vi "bootfile.vi"(11 "parameter file":path=path "D:/dsp files/base_config.set") -> ()   [LabVIEW 2016]
doc: "bootfile.VI connects to the Pixie4 and loads the chosen DSP file. Due to PRIME Lab using 2 PXI crates, the crate size and slot # will need to be adjusted to attain the proper PCI bus address."
uses:
  controls/pixie crates.ctl
  bootfile states.ctl
panel:
  in  "Select PXI chassis type":T1=enum."18-slot chassis"
  in  "Total number of Pixie-4 modules":u16=1
  in  "Slot(s) of Pixie4":u16[](array[numeric])=[8]
  in  "Set":bool
  # "2017.06.01 Note: The Pixie4 is in slot 3 of an 8-slot chassis, but PRIME Lab uses two PXI crates daisy-chained together and XIA's Pixie_Scan_Crate_Slots can't handle multi-crate systems.  Slot 8 of an 18-slot chassis has the same PCI bus and device numbers as Slot 3 of the 1st crate of a two PXI-crate system."
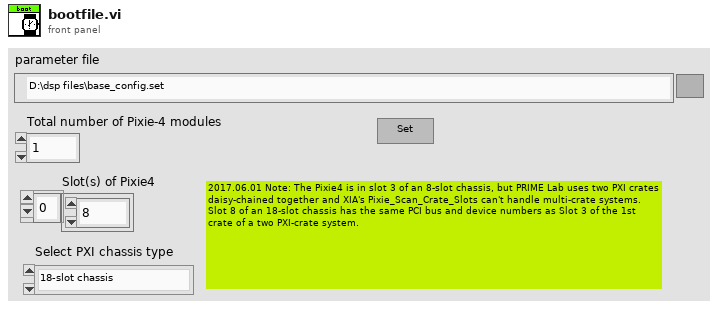
[diagram p1: front panel]
types:
  T1 = typedef "pixie crates.ctl" = enum16{"4 or 8-slot chassis", "14-slot chassis", "18-slot chassis"}
  T2 = typedef "bootfile states.ctl" = enum16{"wait", "set", "stop"}
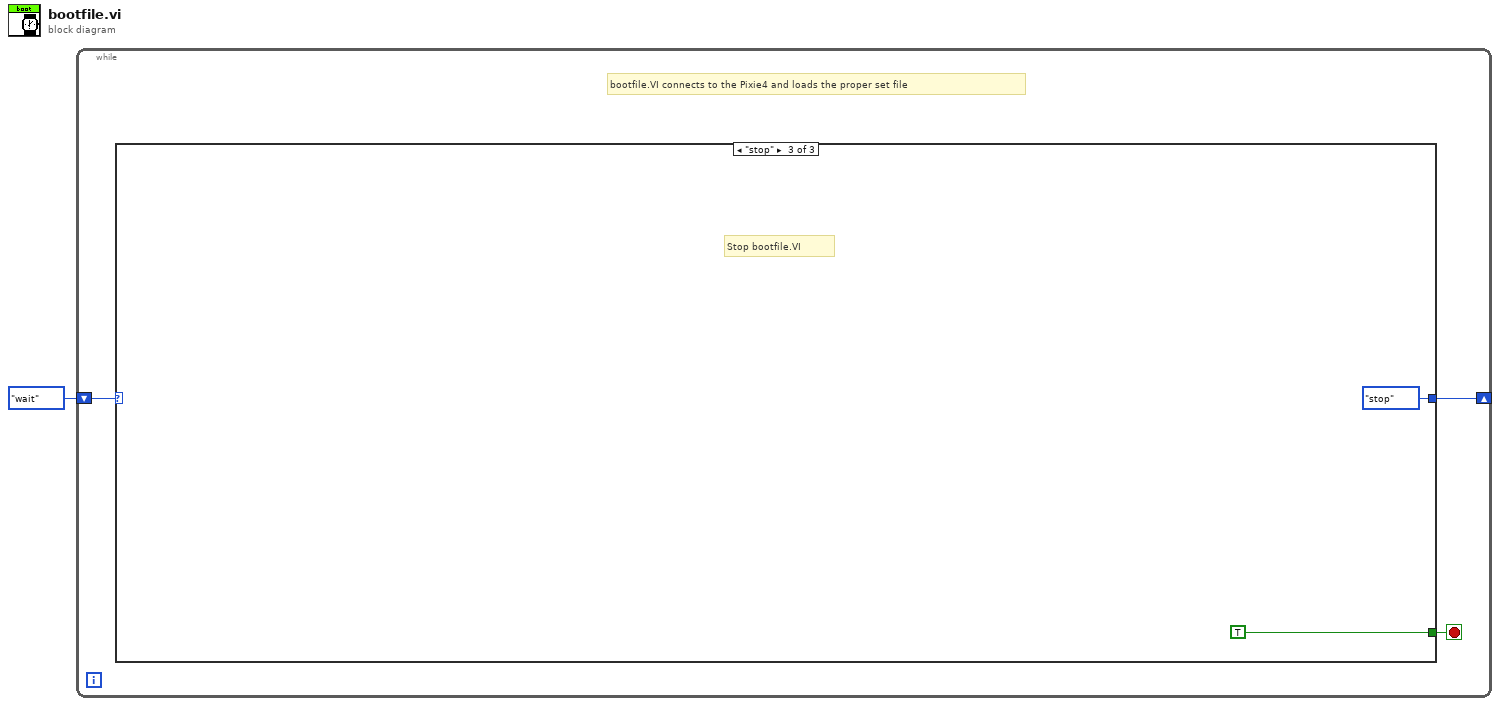
[diagram p0: block diagram]
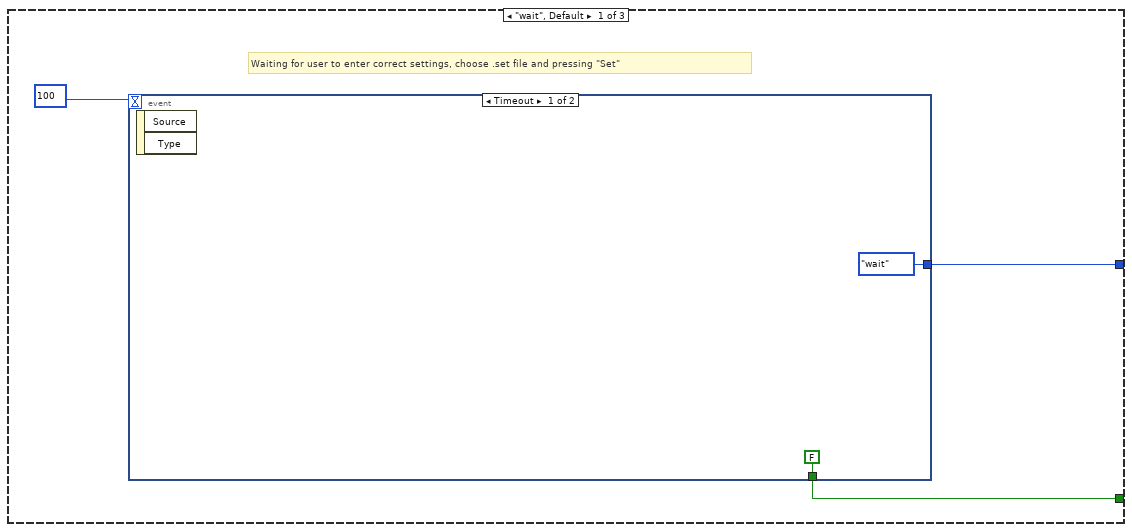
[diagram p2: hidden frame]
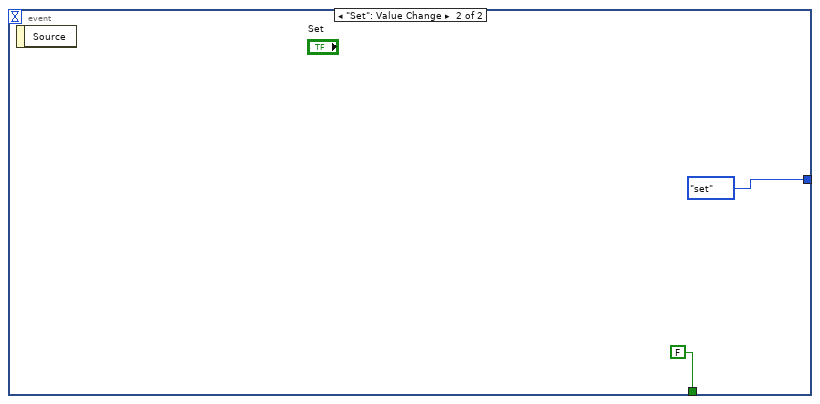
[diagram p3: hidden frame]
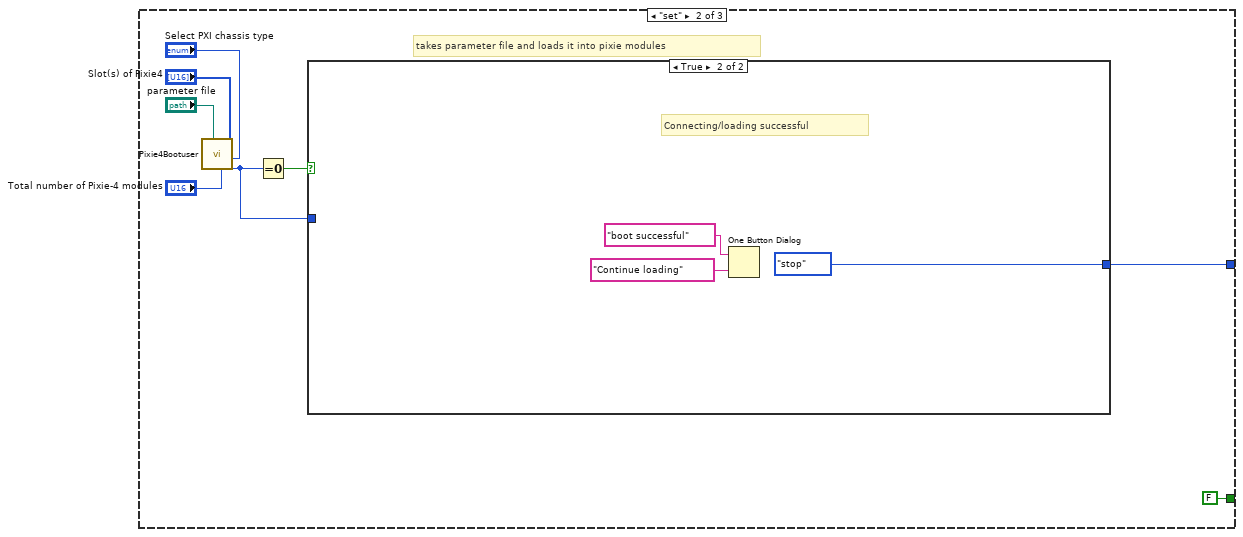
[diagram p4: hidden frame]
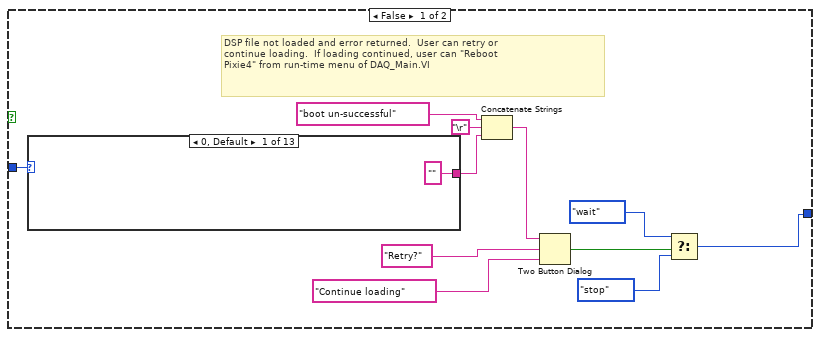
[diagram p5: hidden frame]
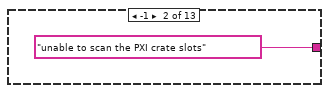
[diagram p6: hidden frame]
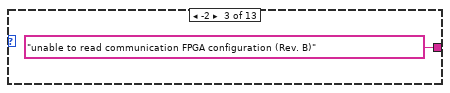
[diagram p7: hidden frame]
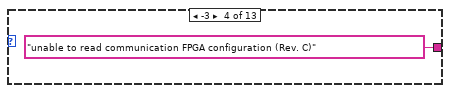
[diagram p8: hidden frame]
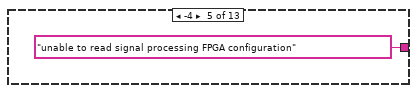
[diagram p9: hidden frame]
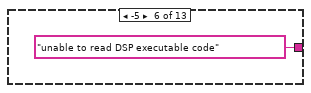
[diagram p10: hidden frame]
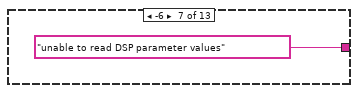
[diagram p11: hidden frame]
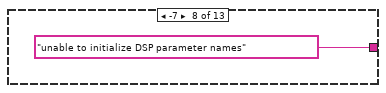
[diagram p12: hidden frame]
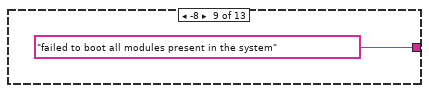
[diagram p13: hidden frame]
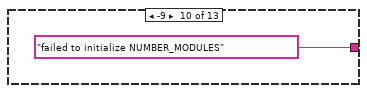
[diagram p14: hidden frame]
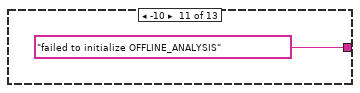
[diagram p15: hidden frame]
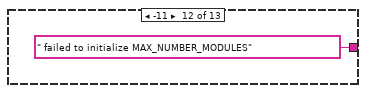
[diagram p16: hidden frame]
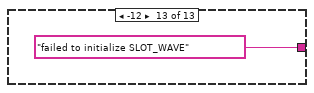
[diagram p17: hidden frame]
diagram:
  n1 = while {
    shift-right: [w2] -> _
    shift-left: bootfile_states."wait" -> [w3]
    stop <- w4 stop-if-true
    # "bootfile.VI connects to the Pixie4 and loads the proper set file"
    n2 = case shown="\"stop\"" w3 {
      tunnel: [w7 FALSE TRUE] -> w4
      tunnel: [w6 w14 bootfile_states."stop"] -> w2
      frame "wait", Default {
        # "Waiting for user to enter correct settings, choose .set file and pressing \"Set\""
        n3 = event shown="[0] Timeout" {
          selector: _ -> [_ _]
          dyn-events: _ -> [_ _]
          timeout: 100 -> [_ _]
          tunnel: [FALSE FALSE] -> w7
          tunnel: [bootfile_states."wait" bootfile_states."set"] -> w6
          event Timeout {
            n4 = event-data() -> ()  [unwired: 1 in, 2 out]
          }
          event "Set": Value Change {
            n5 = event-data() -> ()  [unwired: 1 in, 1 out]
          }
        }
      }
      frame "set" {
        # "takes parameter file and loads it into pixie modules"
        n6 = call "Pixie4Bootuser.vi"("Select PXI chassis type"="Select PXI chassis type", "Module #"="Slot(s) of Pixie4", "Total number of Pixie-4 modules"="Total number of Pixie-4 modules", "DSP parameters file (.set file in folder \"Configuration\")"="parameter file") -> ("Return value for booting"=w13:i32)  [unwired: 7 in]
        n7 = Equal To 0?(x=w13) -> (x = 0?=w15:bool)
        n8 = case shown="True" w15 {
          tunnel: [w22 bootfile_states."stop"] -> w14
          tunnel: w13 -> [w27 _]
          frame False {
            # "DSP file not loaded and error returned.  User can retry or \ncontinue loading.  If loading continued, user can \"Reboot\nPixie4\" from run-time menu of DAQ_Main.VI"
            n9 = case shown="0, Default" w27 {
              tunnel: ["" ("format string") "unable to scan the PXI crate slots" ("format string") "unable to read communication FPGA configuration (Rev. B)" ("format string") "unable to read communication FPGA configuration (Rev. C)" ("format string") "unable to read signal processing FPGA configuration" ("format string") "unable to read DSP executable code" ("format string") "unable to read DSP parameter values" ("format string") "unable to initialize DSP parameter names" ("format string") "failed to boot all modules present in the system" ("format string") "failed to initialize NUMBER_MODULES" ("format string") "failed to initialize OFFLINE_ANALYSIS" ("format string") " failed to initialize MAX_NUMBER_MODULES" ("format string") "failed to initialize SLOT_WAVE" ("format string")] -> w28
              frame 0, Default {
              }
              frame -1 {
              }
              frame -2 {
              }
              frame -3 {
              }
              frame -4 {
              }
              frame -5 {
              }
              frame -6 {
              }
              frame -7 {
              }
              frame -8 {
              }
              frame -9 {
              }
              frame -10 {
              }
              frame -11 {
              }
              frame -12 {
              }
            }
            n10 = Concatenate Strings("boot un-successful" ("format string"), "\r", w28) -> (w26:string)
            n11 = Two Button Dialog(message=w26, 1:"Continue loading" ("F button name (\"Cancel\")"), 2:"Retry?" ("T button name (\"OK\")")) -> (T button?=w23:bool)
            n12 = Select(t=bootfile_states."wait", s=w23, f=bootfile_states."stop") -> (s? t:f=w22:T2)
          }
          frame True {
            # "Connecting/loading successful"
            n13 = One Button Dialog(message="boot successful" ("format string"), button name ("OK")="Continue loading") -> ()  [unwired: 1 out]
          }
        }
      }
      frame "stop" {
        # "Stop bootfile.VI"
      }
    }
  }
